vi "ReceiveSpringDamper.vi"(5 "SpringDamper Input":T1, 6 "Timeout ms":i32=1, 7 "UDP Input":T2) -> (0 "Error Out":errorcluster, 1 "SpringDamper Output":T1, 2 "Did Receive":bool, 3 "UDP Output":T2)   [LabVIEW 2016]
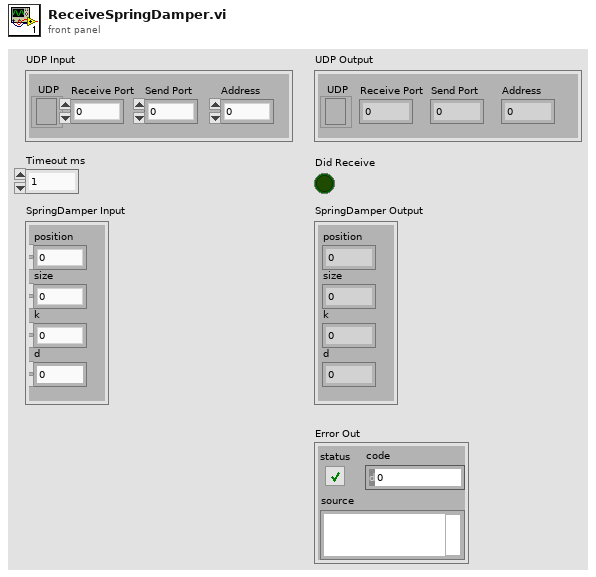
[diagram p1: front panel]
types:
  T1 = cluster{"position":dbl, "size":dbl, "k":dbl, "d":dbl}
  T2 = cluster{"UDP":refnum<k16>, "Receive Port":i32, "Send Port":i32, "Address":i64}
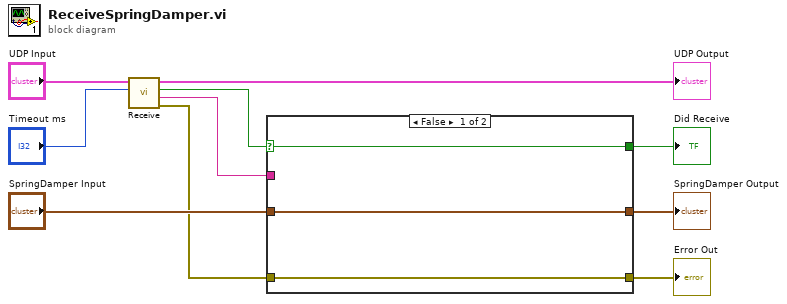
[diagram p0: block diagram]
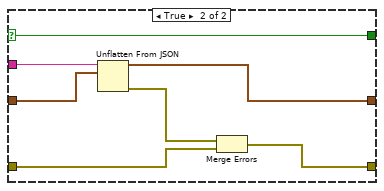
[diagram p2: hidden frame]
diagram:
  n1 = call "Receive.vi"("Timeout ms"="Timeout ms", "UDP Input"="UDP Input") -> ("Error Out"=w5:errorcluster, "Received Data"=w1:string, "Did Receive"=w3:bool, "UDP Output"=→"UDP Output":T2)  [unwired: 2 in]
  n2 = case shown="False" w3 {
    selector: w3 -> [w11 w15]
    tunnel: "SpringDamper Input" -> [w13 w20]
    tunnel: [w12 w18] -> w4
    tunnel: [w13 w19] -> w6
    tunnel: w5 -> [w12 w16]
    tunnel: [w11 w15] -> w2
    tunnel: w1 -> [_ w14]
    frame False {
    }
    frame True {
      n3 = Unflatten From JSON(JSON string=w14, type and defaults=w20) -> (value=w19:T1, error out=w17:errorcluster)  [unwired: 5 in]
      n4 = Merge Errors(w17, w16) -> (w18:errorcluster)
    }
  }
  "Error Out" <- w4
  "SpringDamper Output" <- w6
  "Did Receive" <- w2
